vi "MH_BufferRecordV3.vi"(6 "WindowWidth":i32, 7 "truetime":u64, 8 "WinIndex":i32, 9 "Buffindex":i32, 11 "Buffer":u64[](array[numeric])) -> (0 "WinIndexOut":i32, 1 "BuffIndexOut":i32, 2 "NewBuffsize":i32, 3 "tableau (n rotations)":u64[](array[numeric]), 4 "WindowDelta":i32)   [LabVIEW 2019]
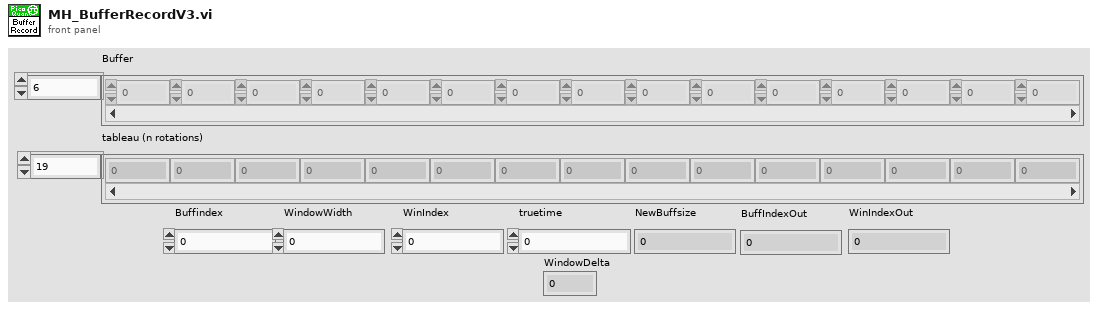
[diagram p1: front panel]
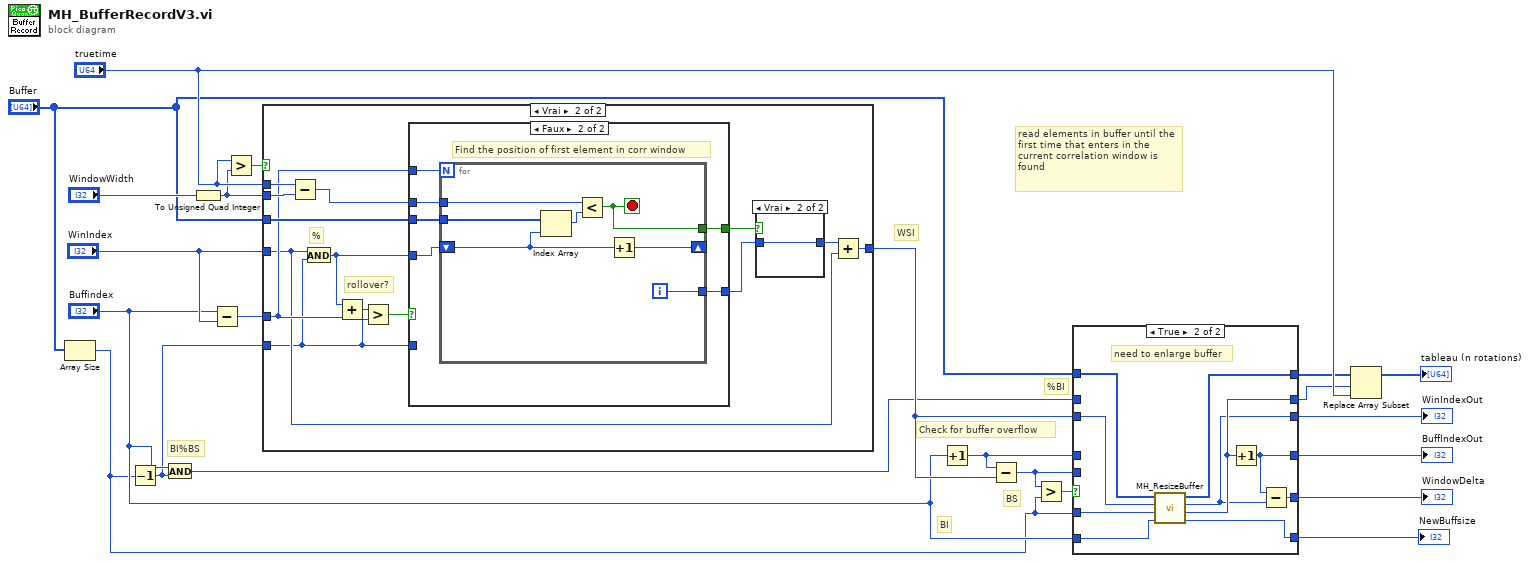
[diagram p0: block diagram]
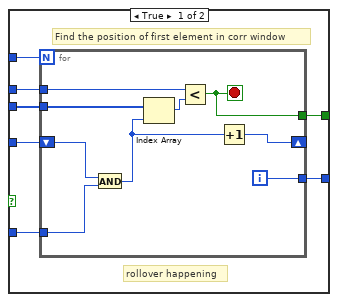
[diagram p3: hidden frame]
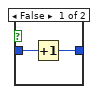
[diagram p4: hidden frame]
diagram:
  # "read elements in buffer until the first time that enters in the current correlation window is found"
  # "BI%BS"
  # "%BI"
  # "BS"
  # "Check for buffer overflow"
  # "WSI"
  # "BI"
  n1 = Array Size(array="Buffer") -> (size(s)=w2:i32)
  n2 = Decrement(x=w2) -> (x-1=w7:i32)
  n3 = And(x="Buffindex", y=w7) -> (x .and. y?=w13:i32)
  n4 = To Unsigned Quad Integer(1:"WindowWidth") -> (0:w6:u64)
  n5 = Subtract(x="Buffindex", y="WinIndex") -> (x-y=w4:i32)
  n6 = Greater?(x="truetime", y=w6) -> (0:w5:bool)
  n7 = case shown="Vrai" w5 {
    tunnel: "Buffer" -> [_ w37]
    tunnel: [w23 w36] -> w16
    tunnel: "WinIndex" -> [w23 w27]
    tunnel: "truetime" -> [_ w35]
    tunnel: w6 -> [_ w34]
    tunnel: w4 -> [_ w30]
    tunnel: w7 -> [_ w25]
    frame False {
      # "this is the case when t<corr window width"
      # "All records will be in window"
    }
    frame True {
      # "rollover?"
      # "%"
      n8 = Subtract(x=w35, y=w34) -> (x-y=w33:u64)
      n9 = And(x=w27, y=w25) -> (x .and. y?=w26:i32)
      n10 = Add(x=w26, y=w30) -> (x+y=w29:i32)
      n11 = Greater?(x=w29, y=w25) -> (0:w24:bool)
      n12 = case shown="Faux" w24 {
        tunnel: w37 -> [w44 w59]
        tunnel: w33 -> [w43 w58]
        tunnel: [w42 w57] -> w32
        tunnel: w30 -> [w41 w56]
        tunnel: [w40 w55] -> w28
        tunnel: w26 -> [w39 w54]
        tunnel: w25 -> [w38 _]
        frame True {
          # "rollover happening"
          # "Find the position of first element in corr window"
          n13 = for {
            N: w41 -> [_]
            tunnel: w43 -> [w50]
            tunnel: w44 -> [w53]
            shift-right: [w52] -> _
            shift-left: w39 -> [w47]
            tunnel: [w49] -> w42
            tunnel: [w48] -> w40
            tunnel: w38 -> [w46]
            i -> [w48]
            stop <- w49 stop-if-true
            n14 = And(x=w47, y=w46) -> (x .and. y?=w45:i32)
            n15 = Index Array(array=w53, index=w45) -> (element=w51:u64)
            n16 = Less?(x=w50, y=w51) -> (x < y?=w49:bool)
            n17 = Increment(x=w45) -> (x+1=w52:i32)
          }
        }
        frame False {
          # "Find the position of first element in corr window"
          n18 = for {
            N: w56 -> [_]
            tunnel: w58 -> [w63]
            tunnel: w59 -> [w66]
            shift-right: [w65] -> _
            shift-left: w54 -> [w60]
            tunnel: [w62] -> w57
            tunnel: [w61] -> w55
            i -> [w61]
            stop <- w62 stop-if-true
            n19 = Index Array(array=w66, index=w60) -> (element=w64:u64)
            n20 = Less?(x=w63, y=w64) -> (x < y?=w62:bool)
            n21 = Increment(x=w60) -> (x+1=w65:i32)
          }
        }
      }
      n22 = case shown="Vrai" w32 {
        tunnel: w28 -> [w68 w69]
        tunnel: [w67 w69] -> w31
        frame False {
          n23 = Increment(x=w68) -> (x+1=w67:i32)
        }
        frame True {
        }
      }
      n24 = Add(x=w31, y=w27) -> (x+y=w36:i32)
    }
  }
  n25 = Increment(x="Buffindex") -> (x+1=w14:i32)
  n26 = Subtract(x=w14, y=w16) -> (x-y=w3:i32)
  n27 = Greater?(x=w3, y=w2) -> (0:w1:bool)
  n28 = case shown="Faux" w1 {
    tunnel: "Buffer" -> [w73 w85]
    tunnel: w2 -> [w74 w82]
    tunnel: [w73 w84] -> w17
    tunnel: "Buffindex" -> [_ w83]
    tunnel: w16 -> [w75 w81]
    tunnel: [w72 w79] -> w15
    tunnel: [w75 w77] -> w18
    tunnel: w13 -> [w72 _]
    tunnel: w14 -> [w71 _]
    tunnel: [w74 w80] -> w9
    tunnel: [w71 w78] -> w12
    tunnel: w3 -> [w70 _]
    tunnel: [w70 w76] -> w8
    frame False {
    }
    frame True {
      # "need to enlarge buffer"
      n29 = call <userlib>:"MH_ResizeBuffer.vi"("Buffindex"=w83, "Buffsize"=w82, "WinIndex"=w81, "Tableau"=w85) -> ("NewBuffsize"=w80:i32, "NewBuffIndex"=w79:i32, "NewWinIndex"=w77:i32, "tableau (n rotations)"=w84:u64[])  [unwired: 2 in, 2 out]
      n30 = Increment(x=w79) -> (x+1=w78:i32)
      n31 = Subtract(x=w78, y=w77) -> (x-y=w76:i32)
    }
  }
  "BuffIndexOut" <- w12
  "WinIndexOut" <- w18
  "NewBuffsize" <- w9
  "WindowDelta" <- w8
  n32 = Replace Array Subset(array=w17, new element="truetime", index=w15) -> (→"tableau (n rotations)":u64[])
